vi "Get Axes Status.vi"(8 "error in (no error)":errorcluster, 10 "Array of axes":T1[](array[typedef]), 11 "VISA in":refnum<visa-resource-name>) -> (0 "error out":errorcluster, 2 "Array of status strings":string[](array[string]), 3 "VISA out":refnum<visa-resource-name>)   [LabVIEW 2018, in "ASI TG-1000.lvlib"]
doc: "Queries the ASI controller for the current position of the specified axes; the equivalent of the WHERE command."
uses:
  ASI TG-1000.lvlib
  Utility/Axis Name.ctl
  Utility/Serial Response Syntax.ctl
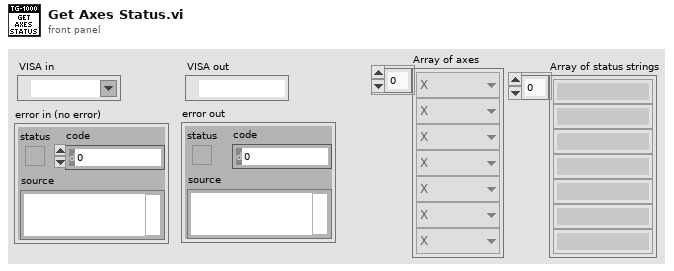
[diagram p1: front panel]
types:
  T1 = typedef "ASI TG-1000.lvlib/Axis Name.ctl" = enum8{"undefined", "A", "B", "C", "D", "E", "F", "G", "H", "I", "J", "K", "L", "M", "N", "O", "P", "Q", "R", "S", "T", "U", "V", "W", "X", "Y", "Z"}
  T2 = typedef "ASI TG-1000.lvlib/Serial Response Syntax.ctl" = enum16{":A then single line", "Single line, no :A", ":A or : then single line", ":A then single number", ":A or : then single number", ":A then <axis>= single number"}
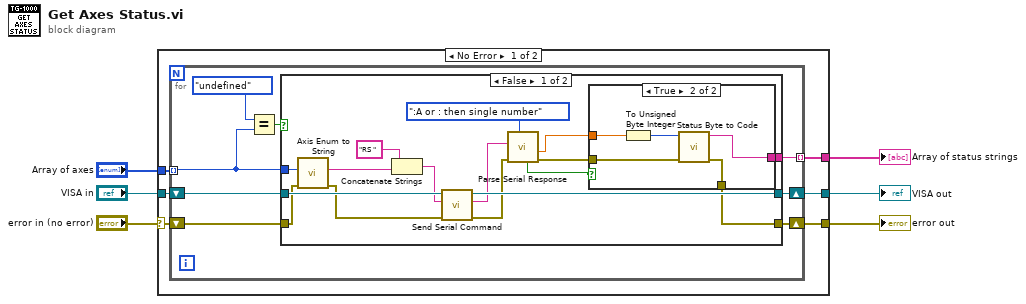
[diagram p0: block diagram]
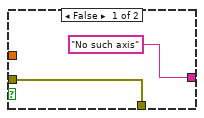
[diagram p2: hidden frame]
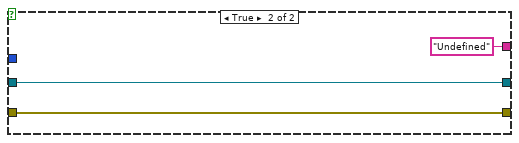
[diagram p3: hidden frame]
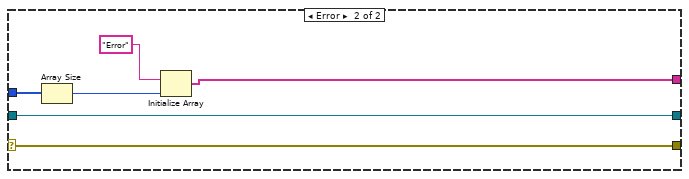
[diagram p4: hidden frame]
diagram:
  n1 = case shown="No Error" "error in (no error)" {
    selector: "error in (no error)" -> [w8 w52]
    tunnel: "VISA in" -> [w12 w51]
    tunnel: [w11 w51] -> w5
    tunnel: [w10 w52] -> w4
    tunnel: "Array of axes" -> [w9 w50]
    tunnel: [w7 w47] -> w1
    frame No Error {
      n2 = for {
        shift-right: [w19] -> w11
        shift-left: w12 -> [w20]
        shift-right: [w16] -> w10
        shift-left: w8 -> [w17]
        tunnel: w9 -> [w14] mode=indexing
        tunnel: [w18] -> w7 mode=indexing
        n3 = Equal?(x=Axis_Name."undefined", y=w14) -> (x = y?=w15:bool)
        n4 = case shown="False" w15 {
          tunnel: w20 -> [w36 w45]
          tunnel: [w35 w45] -> w19
          tunnel: w14 -> [w30 _]
          tunnel: [w27 "Undefined" ("Status Code")] -> w18
          tunnel: w17 -> [w26 w44]
          tunnel: [w23 w44] -> w16
          frame False {
            n5 = call "Axis Enum to String.vi"("error in (no error)"=w26, "Axis Enum In"=w30) -> ("error out"=w25:errorcluster, "Axis String Out"=w29:string)  [unwired: 8 in]
            n6 = Concatenate Strings("RS " ("Command"), w29) -> (w33:string)
            n7 = call "Send Serial Command.vi"("error in (no error)"=w25, "Command"=w33, "VISA in"=w36) -> ("error out"=w28:errorcluster, "Response"=w31:string, "VISA out"=w35:refnum<visa-resource-name>)  [unwired: 6 in]
            n8 = call "Parse Serial Response.vi"("Response Syntax"=Serial_Response_Syntax.":A or : then single number" ("Type of Response"), "error in (no error)"=w28, "Raw Response"=w31) -> ("error out"=w24:errorcluster, "Parsed Double"=w21:dbl, "As expected?"=w22:bool)  [unwired: 5 in, 1 out]
            n9 = case shown="True" w22 {
              tunnel: ["No such axis" ("Status Code") w43] -> w27
              tunnel: w24 -> [w37 w41]
              tunnel: [w37 w40] -> w23
              tunnel: w21 -> [_ w39]
              frame False {
              }
              frame True {
                n10 = To Unsigned Byte Integer(number=w39) -> (unsigned 8bit integer=w42:u8)
                n11 = call "Status Byte to Code.vi"("error in (no error)"=w41, "Status byte [U8]"=w42) -> ("error out"=w40:errorcluster, "Status Code"=w43:string)  [unwired: 8 in]
              }
            }
          }
          frame True {
          }
        }
      }
    }
    frame Error {
      n12 = Array Size(array=w50) -> (size(s)=w49:i32)
      n13 = Initialize Array("Error", w49) -> (w47:string[])
    }
  }
  "VISA out" <- w5
  "error out" <- w4
  "Array of status strings" <- w1
